vi "Write SequencerInfo.vi"(8 "error in (no error)":errorcluster, 10 "Sequencer.lvlib:SequencerInfo.lvclass":refnum<class "SequencerInfo.lvclass">, 11 "Sequencer in":refnum<class "Sequencer.lvclass">) -> (0 "error out":errorcluster, 3 "Sequencer out":refnum<class "Sequencer.lvclass">)   [LabVIEW 2015, in "Sequencer.lvlib" / "Sequencer.lvclass"]
uses:
  Sequencer.lvclass
  SequencerInfo.lvclass
  Sequencer.lvclass/Sequencer.ctl
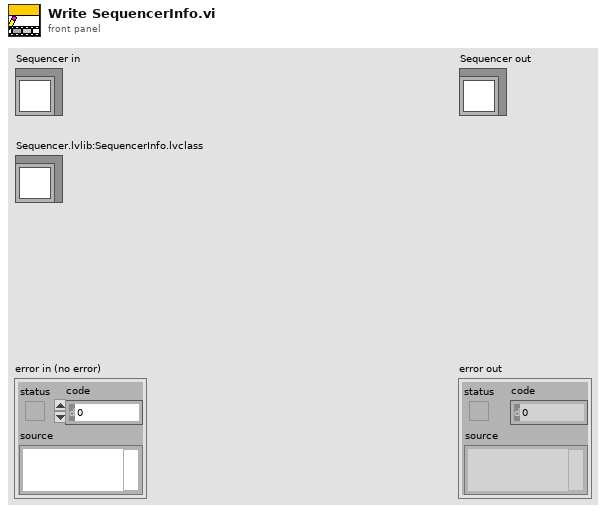
[diagram p1: front panel]
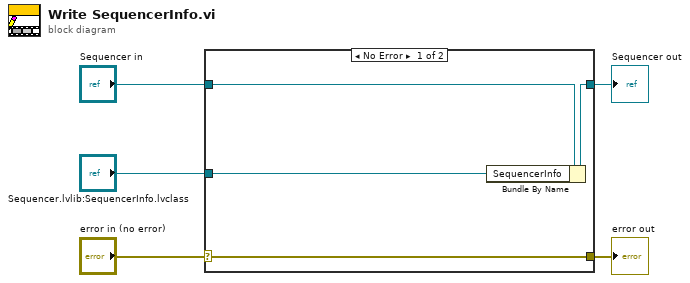
[diagram p0: block diagram]
diagram:
  n1 = case shown="No Error" "error in (no error)" {
    selector: "error in (no error)" -> [w9 w10]
    tunnel: [w9 w10] -> w4
    tunnel: [w7 w11] -> w2
    tunnel: "Sequencer in" -> [w8 w11]
    tunnel: "Sequencer.lvlib:SequencerInfo.lvclass" -> [w6 _]
    frame No Error {
      n2 = Bundle By Name(cluster=w8, "SequencerInfo"=w6) -> (w7:refnum<class "Sequencer.lvclass">)
    }
    frame Error {
    }
  }
  "error out" <- w4
  "Sequencer out" <- w2
